vi "seno.vi"(3 "output control":T1, 4 "data":variant, 5 "X":dbl[](array[numeric]), 6 "a":dbl[](array[numeric])) -> (0 "error out":errorcluster, 1 "f'(X,a)":dbl[][](array[numeric]), 2 "f(X,a)":dbl[](array[numeric]))   [LabVIEW 2023]
doc: "This template is the starting point for creating a model function to be passed to the Nonlinear Curve Fit.vi."
uses:
  <vilib>/gmath/NumericalOptimization/LM_output select.ctl
  <vilib>/gmath/NI_Gmath.lvlib
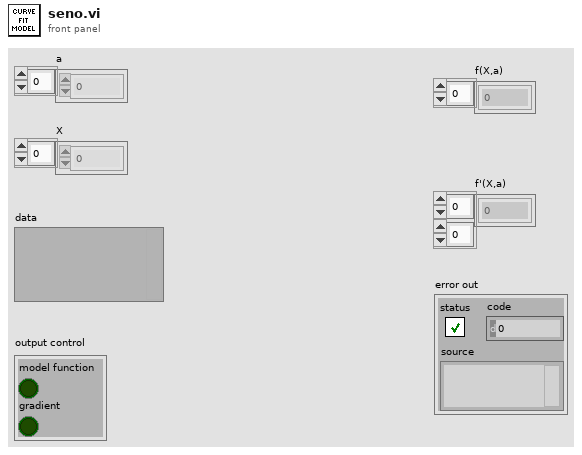
[diagram p1: front panel]
types:
  T1 = typedef "NI_Gmath.lvlib/LM_output select.ctl" = cluster{"model function":bool, "gradient":bool}
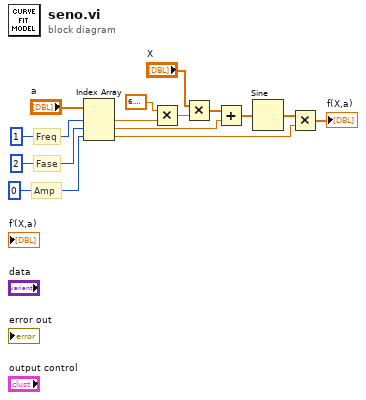
[diagram p0: block diagram]
diagram:
  # "Amp"
  # "Fase"
  # "Freq"
  n1 = Index Array(array="a", index #1=1 ("index"), index #2=2 ("index"), index #3=0 ("index")) -> (element #1=w10:dbl, element #2=w8:dbl, element #3=w5:dbl)
  n2 = Multiply(x=6.283185307179586, y=w10) -> (x*y=w11:dbl)
  n3 = Multiply(x="X", y=w11) -> (x*y=w7:dbl[])
  n4 = Add(x=w7, y=w8) -> (x+y=w6:dbl[])
  n5 = Sine(x=w6) -> (sin(x)=w4:dbl[])
  n6 = Multiply(x=w4, y=w5) -> (x*y=→"f(X,a)":dbl[])
